vi "Import EVT file.vi"(4 "error in (no error)":errorcluster caption="에러 입력(에러 없음)", 7 "file path":path caption="파일 경로") -> (0 "error out":errorcluster caption="에러 출력", 1 "Selected":T1 {"Summary"."Amplitude (selected)" format="%0.2f"}, 2 "Total":T2 {"Summary"."Amplitude (total)" format="%0.2f"}, 3 "File name":string)   [LabVIEW 2017]
uses:
  <vilib>/Utility/file.llb/Read Delimited Spreadsheet (string).vi
  <vilib>/regexp/Match Regular Expression.xnode
  <vilib>/Analysis/NI_AALBase.lvlib
panel:
  out "Class":i32[](array[numeric])
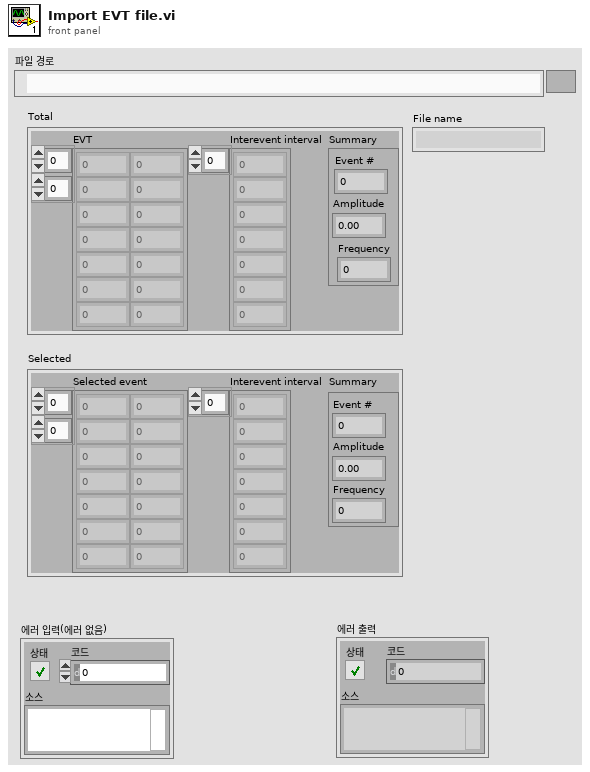
[diagram p1: front panel]
types:
  T1 = cluster{"Selected event":dbl[][], "Interevent interval":dbl[], "Summary":cluster{"Event #":i32, "Amplitude (selected)":dbl, "Frequency":dbl}}
  T2 = cluster{"EVT":dbl[][], "Interevent interval":dbl[], "Summary":cluster{"Event #":i32, "Amplitude (total)":dbl, "Frequency":dbl}}
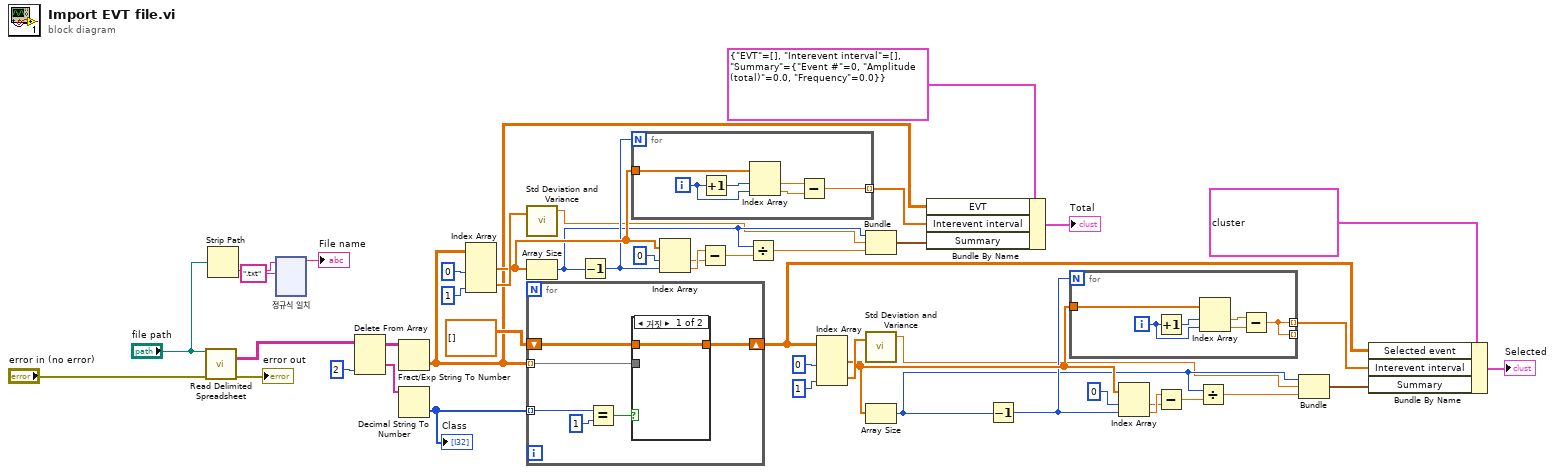
[diagram p0: block diagram]
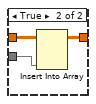
[diagram p2: hidden frame]
diagram:
  n1 = call-poly <vilib>:"Read Delimited Spreadsheet.vi"("file path (dialog if empty)"="file path", "error in (no error)"="error in (no error)") -> ("all rows"=w46:string[][], "error out"=→"error out":errorcluster)  [unwired: 8 in, 4 out]
  n2 = Strip Path(path="file path") -> (name=w3:string)  [unwired: 1 out]
  n3 = xnode "정규식 일치"("입력 문자열"=w3, "정규식"=".txt") -> ("일치 구문 앞"=→"File name":string)  [unwired: 4 in, 4 out]
  n4 = Delete From Array(array=w46, index (col)=2 ("비활성화된 인덱스 (열)")) -> (deleted portion=w44:string[], array with subset deleted=w43:string[][])  [unwired: 2 in]
  n5 = Fract/Exp String To Number(string=w43) -> (number=w19:dbl[][])  [unwired: 3 in, 1 out]
  n6 = Decimal String To Number(string=w44) -> (number=w37:i32[])  [unwired: 2 in, 1 out]
  "Class" <- w37
  n7 = Index Array(array=w19, index (col) #1=0 ("비활성화된 인덱스 (열)"), index (col) #2=1 ("인덱스 (열)")) -> (element #1=w27:dbl[], element #2=w38:dbl[])  [unwired: 2 in]
  n8 = call <vilib>:"Std Deviation and Variance.vi"("X"=w38) -> ("mean"=w16:dbl)  [unwired: 1 in, 2 out]
  n9 = Array Size(array=w27) -> (size(s)=w17:i32)
  n10 = for {
    tunnel: w19 -> [w49] mode=indexing
    tunnel: w37 -> [w52] mode=indexing
    shift-right: [w48] -> w12
    shift-left: dbl[][] [] -> [w47]
    n11 = Equal?(x=w52, y=1) -> (x = y?=w50:bool)
    n12 = case shown="거짓" w50 {
      tunnel: w49 -> [_ w56]
      tunnel: [w53 w55] -> w48
      tunnel: w47 -> [w53 w54]
      frame False {
      }
      frame True {
        n13 = Insert Into Array(array=w54, new element=w56) -> (w55:dbl[][])  [unwired: 2 in]
      }
    }
  }
  n14 = Decrement(x=w17) -> (x-1=w25:i32)
  n15 = for {
    N: w25 -> [_]
    tunnel: w27 -> [w62]
    tunnel: [w57] -> w18 mode=indexing
    i -> [w60]
    n16 = Increment(x=w60) -> (x+1=w61:i32)
    n17 = Index Array(array=w62, index #1=w61, index #2=w60) -> (element #1=w59:dbl, element #2=w58:dbl)
    n18 = Subtract(x=w59, y=w58) -> (x-y=w57:dbl)
  }
  n19 = Index Array(array=w27, index #1=0 ("인덱스"), index #2=w25) -> (element #1=w22:dbl, element #2=w23:dbl)
  n20 = Subtract(x=w23, y=w22) -> (x-y=w21:dbl)
  n21 = Divide(x=w17, y=w21) -> (x/y=w15:dbl)
  n22 = Index Array(array=w12, index (col) #1=0 ("비활성화된 인덱스 (열)"), index (col) #2=1 ("인덱스 (열)")) -> (element #1=w32:dbl[], element #2=w35:dbl[])  [unwired: 2 in]
  n23 = Bundle(w17, "mean"=w16, w15) -> (w14:cluster{i32, "mean":dbl, dbl})  [unwired: 1 in]
  n24 = call <vilib>:"Std Deviation and Variance.vi"("X"=w35) -> ("mean"=w9:dbl)  [unwired: 1 in, 2 out]
  n25 = Array Size(array=w32) -> (size(s)=w10:i32)
  n26 = Bundle By Name(cluster=T2 {"EVT"=[], "Interevent interval"=[], "Summary"={"Event #"=0, "Amplitude (total)"=0.0, "Frequency"=0.0}} ("Total 2"), "EVT"=w19, "Interevent interval"=w18, "Summary"=w14) -> (→"Total":T2)
  n27 = Decrement(x=w10) -> (x-1=w24:i32)
  n28 = for {
    N: w24 -> [_]
    tunnel: w32 -> [w68]
    tunnel: [w63] -> _ mode=indexing
    tunnel: [w63] -> w11 mode=indexing
    i -> [w66]
    n29 = Increment(x=w66) -> (x+1=w67:i32)
    n30 = Index Array(array=w68, index #1=w67, index #2=w66) -> (element #1=w65:dbl, element #2=w64:dbl)
    n31 = Subtract(x=w65, y=w64) -> (x-y=w63:dbl)
  }
  n32 = Index Array(array=w32, index #1=0 ("인덱스"), index #2=w24) -> (element #1=w29:dbl, element #2=w30:dbl)
  n33 = Subtract(x=w30, y=w29) -> (x-y=w28:dbl)
  n34 = Divide(x=w10, y=w28) -> (x/y=w8:dbl)
  n35 = Bundle(w10, "mean"=w9, w8) -> (w7:cluster{i32, "mean":dbl, dbl})  [unwired: 1 in]
  n36 = Bundle By Name(cluster=T1 {"Selected event"=[], "Interevent interval"=[0.05700000000000005, 0.020999999999999963, 0.039000000000000035, 0.01799999999999996, 0.050000000000000044, 0.01200000000000001, 0.028999999999999915, 0.04800000000000004, 0.07899999999999996, 0.08500000000000008, 0.05699999999999994, 0.015000000000000013, 0.031000000000000028, 0.039000000000000035, 0.014999999999999902, 0.07200000000000006, 0.03200000000000003, 0.03299999999999992, 0.08899999999999997, 0.07600000000000007, 0.10000000000000009, 0.07999999999999985, 0.040000000000000036, 0.133, 0.15100000000000002, 0.04800000000000004, 0.08499999999999996, 0.018999999999999906, 0.05300000000000016, 0.16000000000000014, 0.12199999999999989, 0.06999999999999984, 0.038000000000000256, 0.10199999999999987, 0.017999999999999794, 0.08499999999999996, 0.015000000000000124, 0.050000000000000266, 0.08999999999999986, 0.017999999999999794, 0.11800000000000033, 0.054999999999999716, 0.06899999999999995, 0.07299999999999995, 0.013000000000000345, 0.05099999999999971, 0.058000000000000274, 0.008000000000000007, 0.04999999999999982, 0.03100000000000014, 0.05600000000000005, 0.02699999999999969, 0.058000000000000274, 0.08899999999999997, 0.030999999999999694, 0.15500000000000025, 0.020000000000000018, 0.18800000000000017, 0.052999999999999936, 0.02699999999999969, 0.05900000000000016, 0.028999999999999915, 0.019000000000000128, 0.02200000000000024, 0.11499999999999932, 0.1120000000000001, 0.008000000000000007, 0.08400000000000052, 0.11699999999999999, 0.1459999999999999, 0.12399999999999967, 0.014000000000000234, 0.011999999999999567, 0.06100000000000083, 0.0519999999999996, 0.01100000000000012, 0.02799999999999958, 0.07600000000000051, 0.07500000000000018, 0.01699999999999946, 0.08800000000000008, 0.028999999999999915, 0.04800000000000004, 0.06299999999999972, 0.07800000000000029, 0.11099999999999977, 0.10899999999999999, 0.02200000000000024, 0.02800000000000047, 0.1299999999999999, 0.013999999999999346, 0.0990000000000002, 0.03699999999999992, 0.133, 0.028999999999999915, 0.0470000000000006, 0.09899999999999931, 0.08700000000000063, 0.0389999999999997, 0.04499999999999993, 0.04100000000000037, 0.03399999999999981, 0.03200000000000003, 0.0649999999999995, 0.02200000000000024, 0.014000000000000234, 0.14100000000000001, 0.04100000000000037, 0.0029999999999992255, 0.03200000000000003, 0.04600000000000026, 0.04999999999999982, 0.03000000000000025, 0.10099999999999998, 0.038000000000000256, 0.02799999999999958, 0.09600000000000009, 0.04600000000000026, 0.05900000000000016, 0.10999999999999943, 0.0990000000000002, 0.01499999999999968, 0.03000000000000025, 0.04800000000000004, 0.014000000000000234, 0.03399999999999981, 0.006999999999999673, 0.07800000000000029, 0.017999999999999794, 0.17900000000000027, 0.06799999999999962, 0.07699999999999996, 0.11800000000000033, 0.013999999999999346, 0.012000000000000455, 0.062000000000001165, 0.015999999999998238, 0.012000000000000455, 0.0730000000000004, 0.0519999999999996, 0.06300000000000061, 0.015000000000000568, 0.07399999999999984, 0.045999999999999375, 0.09800000000000075, 0.05599999999999916, 0.038000000000000256, 0.129999999999999, 0.04300000000000104, 0.054999999999999716, 0.04800000000000004, 0.04400000000000048, 0.06899999999999906, 0.018000000000000682, 0.06599999999999895, 0.02400000000000091, 0.028999999999999915, 0.04299999999999926, 0.026000000000001577, 0.03399999999999892, 0.12599999999999945, 0.15500000000000114, 0.0259999999999998, 0.12700000000000067, 0.0669999999999984, 0.017000000000001236, 0.1399999999999988, 0.09299999999999997, 0.015000000000000568, 0.021000000000000796, 0.16499999999999915, 0.1379999999999999, 0.10899999999999999, 0.08900000000000041, 0.03599999999999959, 0.03700000000000081, 0.07699999999999996, 0.012000000000000455, 0.16499999999999915, 0.032999999999999474, 0.005000000000000782, 0.07600000000000051, 0.03999999999999915, 0.016000000000000014, 0.013999999999999346, 0.05500000000000149, 0.011999999999998678, 0.014000000000001123, 0.032999999999999474, 0.032999999999999474, 0.053000000000000824, 0.015000000000000568, 0.049999999999998934, 0.019000000000000128, 0.012000000000000455, 0.041999999999999815, 0.09699999999999953, 0.02400000000000091, 0.03500000000000014], "Summary"={"Event #"=0, "Amplitude (selected)"=0.0, "Frequency"=0.0}} ("Selected 2"), "Selected event"=w12, "Interevent interval"=w11, "Summary"=w7) -> (→"Selected":T1)
